vi "burst_count_to_state.vi"(4 "burst count":i32) -> (1 "Burst On":bool)   [LabVIEW 2011]
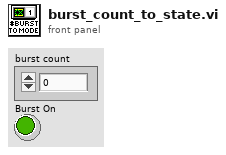
[diagram p1: front panel]
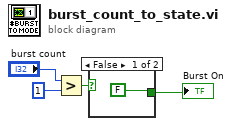
[diagram p0: block diagram]
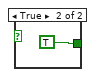
[diagram p2: hidden frame]
diagram:
  n1 = Greater?(x="burst count", y=1) -> (0:w2:bool)
  n2 = case shown="False" w2 {
    tunnel: [FALSE ("Burst") TRUE ("Burst")] -> w1
    frame False {
    }
    frame True {
    }
  }
  "Burst On" <- w1
